vi "FdxCmdTxTrgLineControlCvi.vi"(8 "error in":errorcluster, 9 "TrgLineCtrl":cluster{"TrgInLine":u32, "TrgOutLine":u32} {"TrgInLine" items=["FDX_STROBE_LINE_KEEP"=4294967295, "FDX_STROBE_LINE_OFF"=0, "FDX_STROBE_LINE_1"=1, "FDX_STROBE_LINE_2"=2, "FDX_STROBE_LINE_3"=3, "FDX_STROBE_LINE_4"=4]; "TrgOutLine" items=["FDX_STROBE_LINE_KEEP"=4294967295, "FDX_STROBE_LINE_OFF"=0, "FDX_STROBE_LINE_1"=1, "FDX_STROBE_LINE_2"=2, "FDX_STROBE_LINE_3"=3, "FDX_STROBE_LINE_4"=4]}, 11 "InstrumentHandle_port":u32) -> (0 "error out":errorcluster, 3 "InstrumentHandle_port":u32)   [LabVIEW 2020, in "AIM664LV.lvlib"]
doc: "This function is used to select the Trigger In- and Output lines for the Transmitter part of the associated port. Trigger lines can be used for starting a transmission, or for output of trigger strobes on special frames (especially in the Generic Transmission Mode)."
uses:
  AIM664LV.lvlib
  AFDX_LibraryAdmin/FdxGlobalDllPath.vi
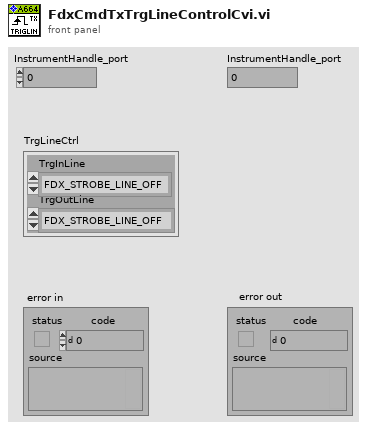
[diagram p1: front panel]
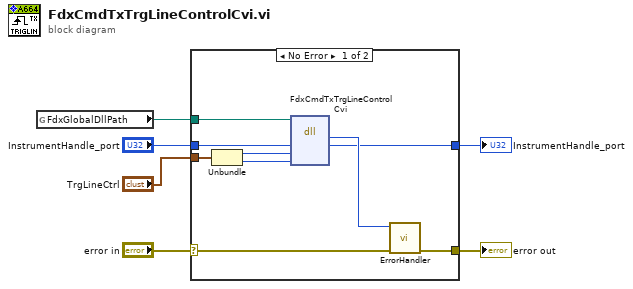
[diagram p0: block diagram]
diagram:
  n1 = global read "FdxGlobalDllPath.vi" "FdxGlobalDllPath"() -> (w4:path)
  n2 = case shown="No Error" "error in" {
    selector: "error in" -> [w14 w17]
    tunnel: [w15 w17] -> w6
    tunnel: w4 -> [w10 _]
    tunnel: "InstrumentHandle_port" -> [w9 w16]
    tunnel: [w8 w16] -> w2
    tunnel: "TrgLineCtrl" -> [w7 _]
    frame No Error {
      n3 = Unbundle(w7) -> ("TrgInLine"=w12:u32, "TrgOutLine"=w11:u32)
      n4 = dll-call lib="aim_fdx.19.dll" fn="FdxCmdTxTrgLineControlCvi"(path in=w10, "InstrumentHandle"=w9, "TrgInLine"=w12, "TrgOutLine"=w11) -> ("status"=w13:i32, "InstrumentHandle"=w8:u32)  [unwired: 4 in, 2 out]
      n5 = call "ErrorHandler.vi"("error in"=w14, "AIM Error"=w13) -> ("error out"=w15:errorcluster)  [unwired: 9 in]
    }
    frame Error {
    }
  }
  "error out" <- w6
  "InstrumentHandle_port" <- w2
